vi "Ranges to Local Points.vi"(11 "Ranges":T3={"Front"=[1.0, 2.0, 3.0, 2.0, 1.0], "Rear"=[1.0, 2.0, 3.0, 2.0, 1.0]}) -> (0 "Rear Range Offset":T1={"X"=-0.27, "Y"=0.0, "Frame"=enum."Local"}, 1 "Front Range Offset":T1={"X"=0.262, "Y"=0.0, "Frame"=enum."Local"}, 2 "Rear Points":T1[](array[typedef]), 3 "Front Points":T1[](array[typedef]))   [LabVIEW 2020, in "FormulaG-Common.lvlib"]
uses:
  FormulaG-Common.lvlib
  Ranges.ctl
  Point.ctl
  Coordinate Frame.ctl
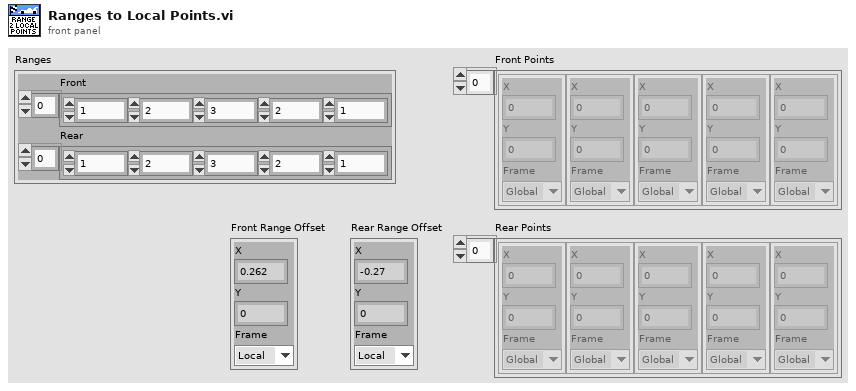
[diagram p1: front panel]
types:
  T1 = typedef "FormulaG-Common.lvlib/Point.ctl" = cluster{"X":sgl, "Y":sgl, "Frame":T2}
  T2 = typedef "FormulaG-Common.lvlib/Coordinate Frame.ctl" = enum16{"Global", "Local"}
  T3 = typedef "FormulaG-Common.lvlib/Ranges.ctl" = cluster{"Front":sgl[], "Rear":sgl[]}
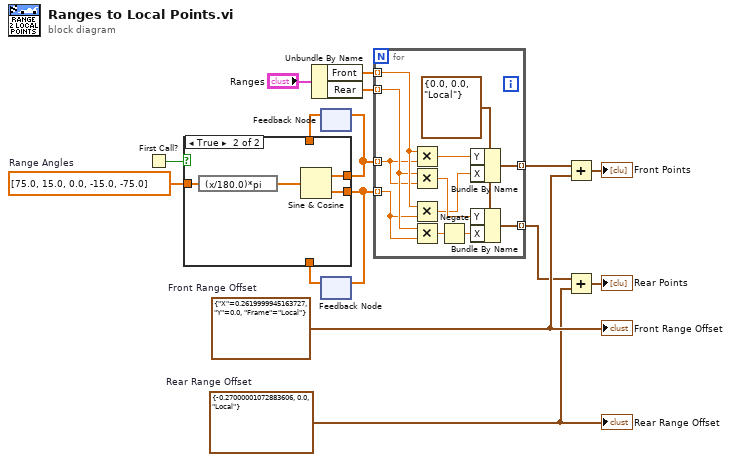
[diagram p0: block diagram]
diagram:
  w3 = T1 {"X"=-0.27, "Y"=0.0, "Frame"=enum."Local"}  # Rear Range Offset
  w5 = T1 {"X"=0.262, "Y"=0.0, "Frame"=enum."Local"}  # Front Range Offset
  w15 = sgl[] [75.0, 15.0, 0.0, -15.0, -75.0]  # Range Angles
  n1 = First Call?() -> (First Call?: T/F=w14:bool)
  n2 = Unbundle By Name("Ranges") -> ("Front"=w10:sgl[], "Rear"=w7:sgl[])
  n3 = feedback #1() -> (w11:sgl[])  [unwired: 1 in]
  n4 = feedback #2() -> (w12:sgl[])  [unwired: 1 in]
  n5 = case shown="True" w14 {
    tunnel: w15 -> [_ w21]
    tunnel: [w17 w19] -> w9
    tunnel: [w16 w18] -> w8
    tunnel: w12 -> [w16 _]
    tunnel: w11 -> [w17 _]
    frame False {
    }
    frame True {
      n6 = expression code="(x/180.0)*pi" ("degrees to radians")(w21) -> (w20:sgl[])
      n7 = Sine & Cosine(0:w20) -> (1:w19:sgl[], 2:w18:sgl[])
    }
  }
  n8 = feedback-in #1(w9) -> ()
  n9 = feedback-in #2(w8) -> ()
  n10 = for {
    tunnel: w10 -> [w33] mode=indexing
    tunnel: w9 -> [w30] mode=indexing
    tunnel: w8 -> [w31] mode=indexing
    tunnel: w7 -> [w32] mode=indexing
    tunnel: [w24] -> w6 mode=indexing
    tunnel: [w23] -> w4 mode=indexing
    w29 = T1 {"X"=0.0, "Y"=0.0, "Frame"=enum."Local"} ("Point")
    n11 = Multiply(x=w33, y=w30) -> (x*y=w28:sgl)
    n12 = Multiply(x=w32, y=w30) -> (x*y=w27:sgl)
    n13 = Multiply(x=w33, y=w31) -> (x*y=w26:sgl)
    n14 = Multiply(x=w32, y=w31) -> (x*y=w25:sgl)
    n15 = Negate(x=w25) -> (-x=w22:sgl)
    n16 = Bundle By Name(cluster=w29, "Y"=w28, "X"=w26) -> (w24:T1)
    n17 = Bundle By Name(cluster=w29, "Y"=w27, "X"=w22) -> (w23:T1)
  }
  n18 = Add(x=w6, y=w5) -> (x+y=→"Front Points":cluster{"X":sgl, "Y":sgl, "Frame":u16}[])
  n19 = Add(x=w4, y=w3) -> (x+y=→"Rear Points":cluster{"X":sgl, "Y":sgl, "Frame":u16}[])
  "Front Range Offset" <- w5
  "Rear Range Offset" <- w3
